vi "RT Driver VI.vi"(7 "Operation":T1, 11 "Device Reference in":T2 format="%.0x") -> (0 "Error Code":i32)   [LabVIEW 2015, in "DMM-SWITCH-ScanList Engine.lvlib"]
uses:
  DMM-SWITCH-ScanList Engine.lvlib
  <vilib>/NI Veristand/Custom Device API/Custom Device Item Ref.ctl
  <vilib>/NI Veristand/Custom Device API/Hardware Interface Driver VI Operation.ctl
  Shared/Compiled.Settings
  TypeDefs/DMM-Switch Configuration.ctl
  <instrlib>/niDMM/nidmm.llb/niDMM Function.ctl
  <instrlib>/niDMM/nidmm.llb/niDMM Resolution in Digits.ctl
  <instrlib>/niSwitch/niSwitch.LLB/niSwitch Topologies.ctl
  <instrlib>/niSwitch/niSwitch.LLB/niSwitch Trigger Input.ctl
  <instrlib>/niSwitch/niSwitch.LLB/niSwitch Scan Advanced Output.ctl
  <instrlib>/niDMM/nidmm.llb/niDMM Measurement Complete.ctl
  <instrlib>/niDMM/nidmm.llb/niDMM Trigger.ctl
  TypeDefs/RTStateVariables.ctl
  <vilib>/addons/Inline Async API/_VS Inline Async API/VS Inline Async API/VS Inline Async API.lvclass
  <vilib>/addons/Inline Async API/_VS Inline Async API/VS Inline Async API/VS Inline Async API.lvclass/VS Inline Async API.ctl
  <vilib>/addons/Inline Async API/_Data Access Engine/Data Access Engine/Data Access Engine.lvclass/Data Access Engine.ctl
  <vilib>/addons/Inline Async API/_Data Access Engine/Access Type Classes/Write/Write.lvclass/Write.ctl
  <vilib>/addons/Inline Async API/_Data Access Engine/Access Type Classes/ReadWrite/ReadWrite.lvclass/ReadWrite.ctl
  <vilib>/addons/Inline Async API/_Data Access Engine/Access Type Classes/Read/Read.lvclass/Read.ctl
  <vilib>/addons/Inline Async API/_Data Access Engine/Data Access Engine/Methods/Data.Engine.Read Data from HW.vi
  <vilib>/addons/Inline Async API/_Data Access Engine/Data Access Engine/Methods/Data.Engine.Write Data to HW.vi
  <vilib>/addons/Inline Async API/_Data Access Engine/Access Type Classes/ReadWrite/ReadWrite.EngineData.vi
  <vilib>/addons/Inline Async API/_Data Access Engine/Access Type Classes/Write/Write.EngineData.vi
  <vilib>/addons/Inline Async API/_Data Access Engine/Access Type Classes/Read/Read.EngineData.vi
  <vilib>/NI Veristand/Custom Device API/NI VeriStand - Get Channel Value by Data Reference.vi
  <vilib>/NI Veristand/Custom Device API/NI VeriStand - Set Channel Value by Data Reference.vi
  <vilib>/NI Veristand/Custom Device API/NI VeriStand - Get Channel Values by Block Data Reference.vi
  <vilib>/NI Veristand/Custom Device API/Global Data Refs.vi
  <vilib>/NI Veristand/Custom Device API/Get Item Property (Variant).vi
  Runtime.Async.vi
  Shared/DMM-SWITCH-ScanList Shared.lvlib
  <vilib>/NI Veristand/Custom Device API/Custom Device API.lvlib
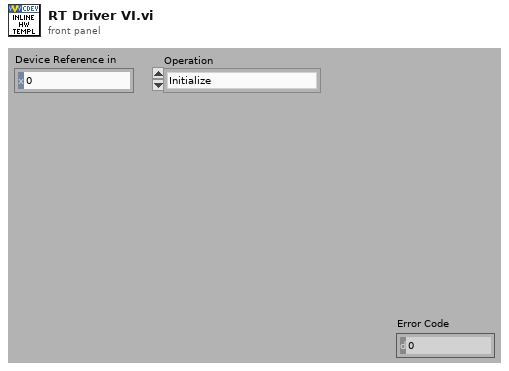
[diagram p1: front panel]
types:
  T1 = typedef "Custom Device API.lvlib/Hardware Interface Driver VI Operation.ctl" = enum16{"Initialize", "Start", "Read Data from HW", "Write Data to HW", "Close"}
  T2 = typedef "Custom Device API.lvlib/Custom Device Item Ref.ctl" = u64
  T3 = typedef "DMM-SWITCH-ScanList Engine.lvlib/RTStateVariables.ctl" = cluster{"Async":refnum<class "VS Inline Async API.lvclass">, "Settings":T4}
  T4 = typedef "DMM-SWITCH-ScanList Shared.lvlib/Compiled.Settings" = cluster{"Name":string, "DMM-Switch Configuration":T5}
  T5 = typedef "DMM-SWITCH-ScanList Engine.lvlib/DMM-Switch Configuration.ctl" = cluster{"DMM Resource Name":string, "DMM Measurement":T6, "DMM Resolution in Digits":T7, "DMM Range [EU]":dbl, "Switch Resource Name":string, "Switch Topology":T8, "Switch Scan List":string, "Switch Trigger Source":T9, "Switch Scan Advanced Output":T10, "DMM Measurement Complete":T11, "DMM Trigger Source":T12, "# of Channels":u32, "Group CH Names - Configuration":string, "Group CH Names - Input Channels":string, "Group CH Names - Measurement Channels":string, "Group CH Names - Runtime Status":string}
  T6 = typedef "niDMM Function.ctl" = enum16{"DC Volts", "AC Volts", "DC Current", "AC Current", "2-wire Resistance", "4-wire Resistance", "Diode", "Frequency", "Period", "AC Volts DC Coupled", "Capacitance", "Inductance", "Temperature"}
  T7 = typedef "niDMM Resolution in Digits.ctl" = dbl
  T8 = typedef "niSwitch Topologies.ctl" = string
  T9 = typedef "niSwitch Trigger Input.ctl" = enum16{"Immediate", "External", "TTL0", "TTL1", "TTL2", "TTL3", "TTL4", "TTL5", "TTL6", "TTL7", "ECL0", "ECL1", "PXI Star", "Software Trigger Function", "Rear Connector", "Front Connector", "Rear Connector of Module 1", "Rear Connector of Module 2", "Rear Connector of Module 3", "Rear Connector of Module 4", "Rear Connector of Module 5", "Rear Connector of Module 6", "Rear Connector of Module 7", "Rear Connector of Module 8", "Rear Connector of Module 9", "Rear Connector of Module 10", "Rear Connector of Module 11", "Rear Connector of Module 12", "Front Connector of Module 1", "Front Connector of Module 2", "Front Connector of Module 3", "Front Connector of Module 4", "Front Connector of Module 5", "Front Connector of Module 6", "Front Connector of Module 7", "Front Connector of Module 8", "Front Connector of Module 9", "Front Connector of Module 10", "Front Connector of Module 11", "Front Connector of Module 12"}
  T10 = typedef "niSwitch Scan Advanced Output.ctl" = enum16{"None", "External", "TTL0", "TTL1", "TTL2", "TTL3", "TTL4", "TTL5", "TTL6", "TTL7", "ECL0", "ECL1", "PXI Star", "Rear Connector", "Front Connector", "Rear Connector Module 1", "Rear Connector Module 2", "Rear Connector Module 3", "Rear Connector Module 4", "Rear Connector Module 5", "Rear Connector Module 6", "Rear Connector Module 7", "Rear Connector Module 8", "Rear Connector Module 9", "Rear Connector Module 10", "Rear Connector Module 11", "Rear Connector Module 12", "Front Connector Module 1", "Front Connector Module 2", "Front Connector Module 3", "Front Connector Module 4", "Front Connector Module 5", "Front Connector Module 6", "Front Connector Module 7", "Front Connector Module 8", "Front Connector Module 9", "Front Connector Module 10", "Front Connector Module 11", "Front Connector Module 12"}
  T11 = typedef "niDMM Measurement Complete.ctl" = enum16{"None", "External", "TTL 0", "TTL 1", "TTL 2", "TTL 3", "TTL 4", "TTL 5", "TTL 6", "TTL 7", "LBR Trig 0"}
  T12 = typedef "niDMM Trigger.ctl" = enum16{"Immediate", "External", "TTL 0", "TTL 1", "TTL 2", "TTL 3", "TTL 4", "TTL 5", "TTL 6", "Software", "TTL 7", "PXI Star", "LBR Trig 1", "Aux Trig 1"}
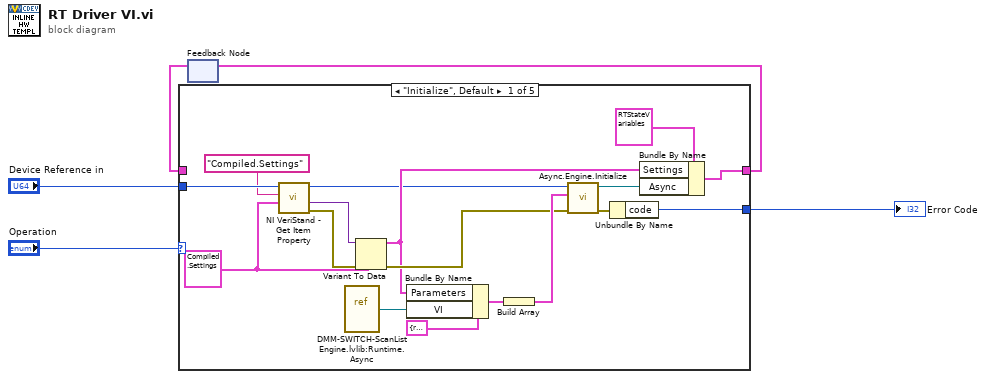
[diagram p0: block diagram]
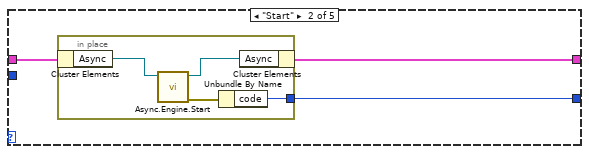
[diagram p2: hidden frame]
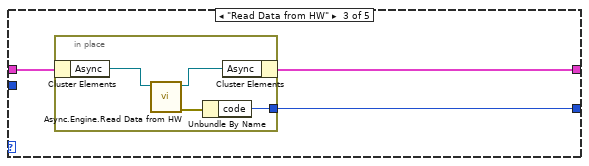
[diagram p3: hidden frame]
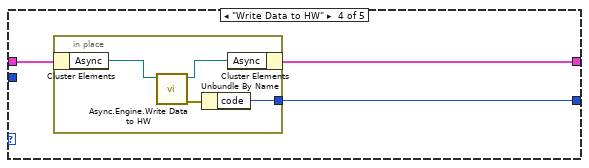
[diagram p4: hidden frame]
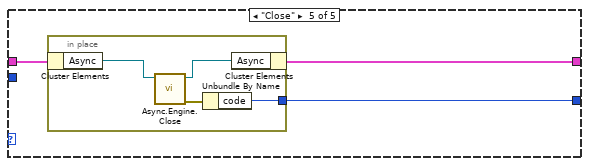
[diagram p5: hidden frame]
diagram:
  n1 = feedback #1() -> (w4:T3)  [unwired: 1 out]
  n2 = case shown="\"Initialize\", Default" "Operation" {
    tunnel: [w20 w24 w30 w37 w45] -> w5
    tunnel: w4 -> [_ w25 w32 w38 w46]
    tunnel: "Device Reference in" -> [w16 _ _ _ _]
    tunnel: [w22 w23 w31 w39 w44] -> w1
    frame "Initialize", Default {
      w12 = T4 {"Name"="", "DMM-Switch Configuration"={"DMM Resource Name"="", "DMM Measurement"=enum."DC Volts", "DMM Resolution in Digits"=6.5, "DMM Range [EU]"=10.0, "Switch Resource Name"="", "Switch Topology"="2503/2-Wire 24x1 Mux", "Switch Scan List"="ab0->com0 & com0->ch0:2;", "Switch Trigger Source"=enum."TTL0", "Switch Scan Advanced Output"=enum."TTL1", "DMM Measurement Complete"=enum."TTL 0", "DMM Trigger Source"=enum."TTL 1", "# of Channels"=0, "Group CH Names - Configuration"="", "Group CH Names - Input Channels"="", "Group CH Names - Measurement Channels"="", "Group CH Names - Runtime Status"=""}}
      n3 = call-poly <vilib>:"NI VeriStand - Get Item Property.vi"("Default Value"=w12, "Property Name"="Compiled.Settings", "Item Ref in"=w16) -> ("error out"=w15:errorcluster, "Value"=w14:variant, "Item Ref out"=w8:T2)  [unwired: 5 in, 1 out]
      n4 = vi-ref "DMM-SWITCH-ScanList Engine.lvlib:Runtime.Async.vi"() -> (w18:refnum<vi>)
      n5 = Variant To Data(error in=w15, type=w12, Variant=w14) -> (data=w9:T4, error out=w10:errorcluster)
      n6 = Bundle By Name(cluster=cluster{"VI":refnum<vi>, "Parameters":variant} {"VI"=refnum, "Parameters"=variant} ("Process"), "Parameters"=w9, "VI"=w18) -> (w17:cluster{"VI":refnum<vi>, "Parameters":variant})
      n7 = Build Array(w17) -> (w11:cluster{"VI":refnum<vi>, "Parameters":variant}[])
      n8 = call <vilib>:"Async.Engine.Initialize.vi"("error in (no error)"=w10, "Processes"=w11, "Custom Device Ref"=w8) -> ("error out"=w6:errorcluster, "Async"=w21:refnum<class "VS Inline Async API.lvclass">)  [unwired: 7 in]
      n9 = Unbundle By Name(w6) -> ("code"=w22:i32)
      n10 = Bundle By Name(cluster=T3 {"Async"=refnum, "Settings"={"Name"="", "DMM-Switch Configuration"={"DMM Resource Name"="", "DMM Measurement"=enum."DC Volts", "DMM Resolution in Digits"=6.5, "DMM Range [EU]"=10.0, "Switch Resource Name"="", "Switch Topology"="2503/2-Wire 24x1 Mux", "Switch Scan List"="ab0->com0 & com0->ch0:2;", "Switch Trigger Source"=enum."TTL0", "Switch Scan Advanced Output"=enum."TTL1", "DMM Measurement Complete"=enum."TTL 0", "DMM Trigger Source"=enum."TTL 1", "# of Channels"=0, "Group CH Names - Configuration"="", "Group CH Names - Input Channels"="", "Group CH Names - Measurement Channels"="", "Group CH Names - Runtime Status"=""}}} ("RT State Variables"), "Settings"=w9, "Async"=w21) -> (w20:T3)
    }
    frame "Start" {
      n11 = in-place {
        in-place-border: [w27] -> w23
        n12 = in-place-cluster #2(w25) -> ("Async"=w29:refnum<class "VS Inline Async API.lvclass">)
        n13 = call <vilib>:"Async.Engine.Start.vi"("VS Inline Async API in"=w29) -> ("error out"=w26:errorcluster, "VS Inline Async API out"=w28:refnum<class "VS Inline Async API.lvclass">)  [unwired: 9 in]
        n14 = Unbundle By Name(w26) -> ("code"=w27:i32)
        n15 = in-place-cluster #2("Async"=w28) -> (w24:T3)
      }
    }
    frame "Read Data from HW" {
      n16 = in-place {
        in-place-border: [w34] -> w31
        n17 = in-place-cluster #3(w32) -> ("Async"=w36:refnum<class "VS Inline Async API.lvclass">)
        n18 = call <vilib>:"Async.Engine.Read Data from HW.vi"("Async in"=w36) -> ("error out"=w33:errorcluster, "Async out"=w35:refnum<class "VS Inline Async API.lvclass">)  [unwired: 9 in]
        n19 = Unbundle By Name(w33) -> ("code"=w34:i32)
        n20 = in-place-cluster #3("Async"=w35) -> (w30:T3)
      }
    }
    frame "Write Data to HW" {
      n21 = in-place {
        in-place-border: [w43] -> w39
        n22 = in-place-cluster #4(w38) -> ("Async"=w42:refnum<class "VS Inline Async API.lvclass">)
        n23 = call <vilib>:"Async.Engine.Write Data to HW.vi"("VS Inline Async API in"=w42) -> ("error out"=w40:errorcluster, "VS Inline Async API out"=w41:refnum<class "VS Inline Async API.lvclass">)  [unwired: 9 in]
        n24 = Unbundle By Name(w40) -> ("code"=w43:i32)
        n25 = in-place-cluster #4("Async"=w41) -> (w37:T3)
      }
    }
    frame "Close" {
      n26 = in-place {
        in-place-border: [w48] -> w44
        n27 = in-place-cluster #5(w46) -> ("Async"=w50:refnum<class "VS Inline Async API.lvclass">)
        n28 = call <vilib>:"Async.Engine.Close.vi"("Async in"=w50) -> ("error out"=w47:errorcluster, "Async out"=w49:refnum<class "VS Inline Async API.lvclass">)  [unwired: 9 in]
        n29 = Unbundle By Name(w47) -> ("code"=w48:i32)
        n30 = in-place-cluster #5("Async"=w49) -> (w45:T3)
      }
    }
  }
  "Error Code" <- w1
  n31 = feedback-in #1(w5) -> ()
